vi "Helium Fridge Cool-Down - Copy.vi"() -> ()   [LabVIEW 2014]
uses:
  <vilib>/Analysis/8numeric.llb/1D Numeric Integration.vi
  <vilib>/express/express shared/transition.llb/Dynamic To Waveform Array.vi
  <vilib>/express/express signal manip/GetorSetDDTAttributes/Set DDT Attributes/SetT0.vi
  <vilib>/express/express shared/transition.llb/Waveform Array To Dynamic.vi
  <vilib>/express/express signal manip/GetorSetDDTAttributes/Set DDT Attributes/Set DDT Properties.xnode
  <vilib>/Analysis/NI_AALPro.lvlib
panel:
  out "Session Out 2":refnum<visa-resource-name>
  out "error out 2":errorcluster {"code" format="%.0x"}
  out "token":dbl
  in  "error in 2":errorcluster {"code" format="%.0x"}
  in  "Session In 2":refnum<visa-resource-name>="HPSIGGEN"
  in  "Depth/Div Submit":bool
  out "Depth/Div (kHz)":dbl
  in  "Cent. Frq. Submit":bool
  out "Session Out":refnum<visa-resource-name>
  out "error out":errorcluster {"code" format="%.0x"}
  out "Central Frequency":dbl
  in  "error in":errorcluster {"code" format="%.0x"}
  in  "Session In":refnum<visa-resource-name>="HPSIGGEN"
  out "Cent. Freq. (MHz)":dbl
  out "Temp 2":bool
  out "Temperature Strip Chart":dynamicdata(graph)
  in  "TC Points/Measurement":dbl=20.0
  out "NMR":bool
  out "NMR Temp Error":bool
  out "Q Meter Temp":dynamicdata(graph)
  out "Zeroed Array":dbl[](array[numeric])
  out "Fit X values":dbl[](array[numeric])
  in  "Left wing 2":dbl
  in  "Right wing 2":dbl
  in  "Right wing":dbl
  in  "Left wing":dbl
  out "Fit":dbl[](array[numeric])
  in  "Submit":bool
  out "Is Flashing":bool
  in  "Error Beat":bool
  in  "Clear":bool
  in  "Comment":string
  out "Heartbeat":bool
  out "Most Recent Error":string
  out "Baseline Subtracted Integral vs. Time":dbl(graph)
  out "Time of Last Baseline":string
  out "Baseline":dbl[](array[numeric])
  in  "Baseline Subtract":bool
  in  "Get Baseline":bool
  out "Recording":bool
  out "Time of Last Recording":string
  in  "Record \nNMR Sweeps":bool
  in  "Depth/Div\n(MHz)":dbl=10.0
  in  "Central Freq. \n(MHz)":dbl=13.0
  in  "stop (F)":bool caption="Triangle Wave"
  in  "Triangle Wave\nRate (Hz)":dbl=0.3
  out "Time Elapsed \nDuring Sweeps (s)":dbl
  out "Lab Time":string
  out "Most Recent Error (NMR)":string
  out "Last Sweep Start Time":string
  out "Most Recent Error (Temp)":string
  out "Last Measurement Taken":string
  out "VI Start Time":string
  in  "Time Between\nTemp Ponts (s)":dbl=30.0
  out "Temp":bool
  out "NMR":bool
  in  "stop":bool
  out "Input Triangle Wave":dynamicdata(graph)
  out "Modulator":dynamicdata(graph)
  out "NMR":cluster{"Y":dbl[], "Y":dbl[]}[](graph)
  in  "# of Sweeps":dbl=1.0
  out "Resistance Strip Chart":dynamicdata(graph)
  in  "Heartbeat":bool
  in  "Temp Strip Chart":bool
  out "Errors":bool
  in  "Silence Flashing":bool
  # "Initialization and Logic Controls -- DO NOT TOUCH!!"
  # "Caitlyn's Work"
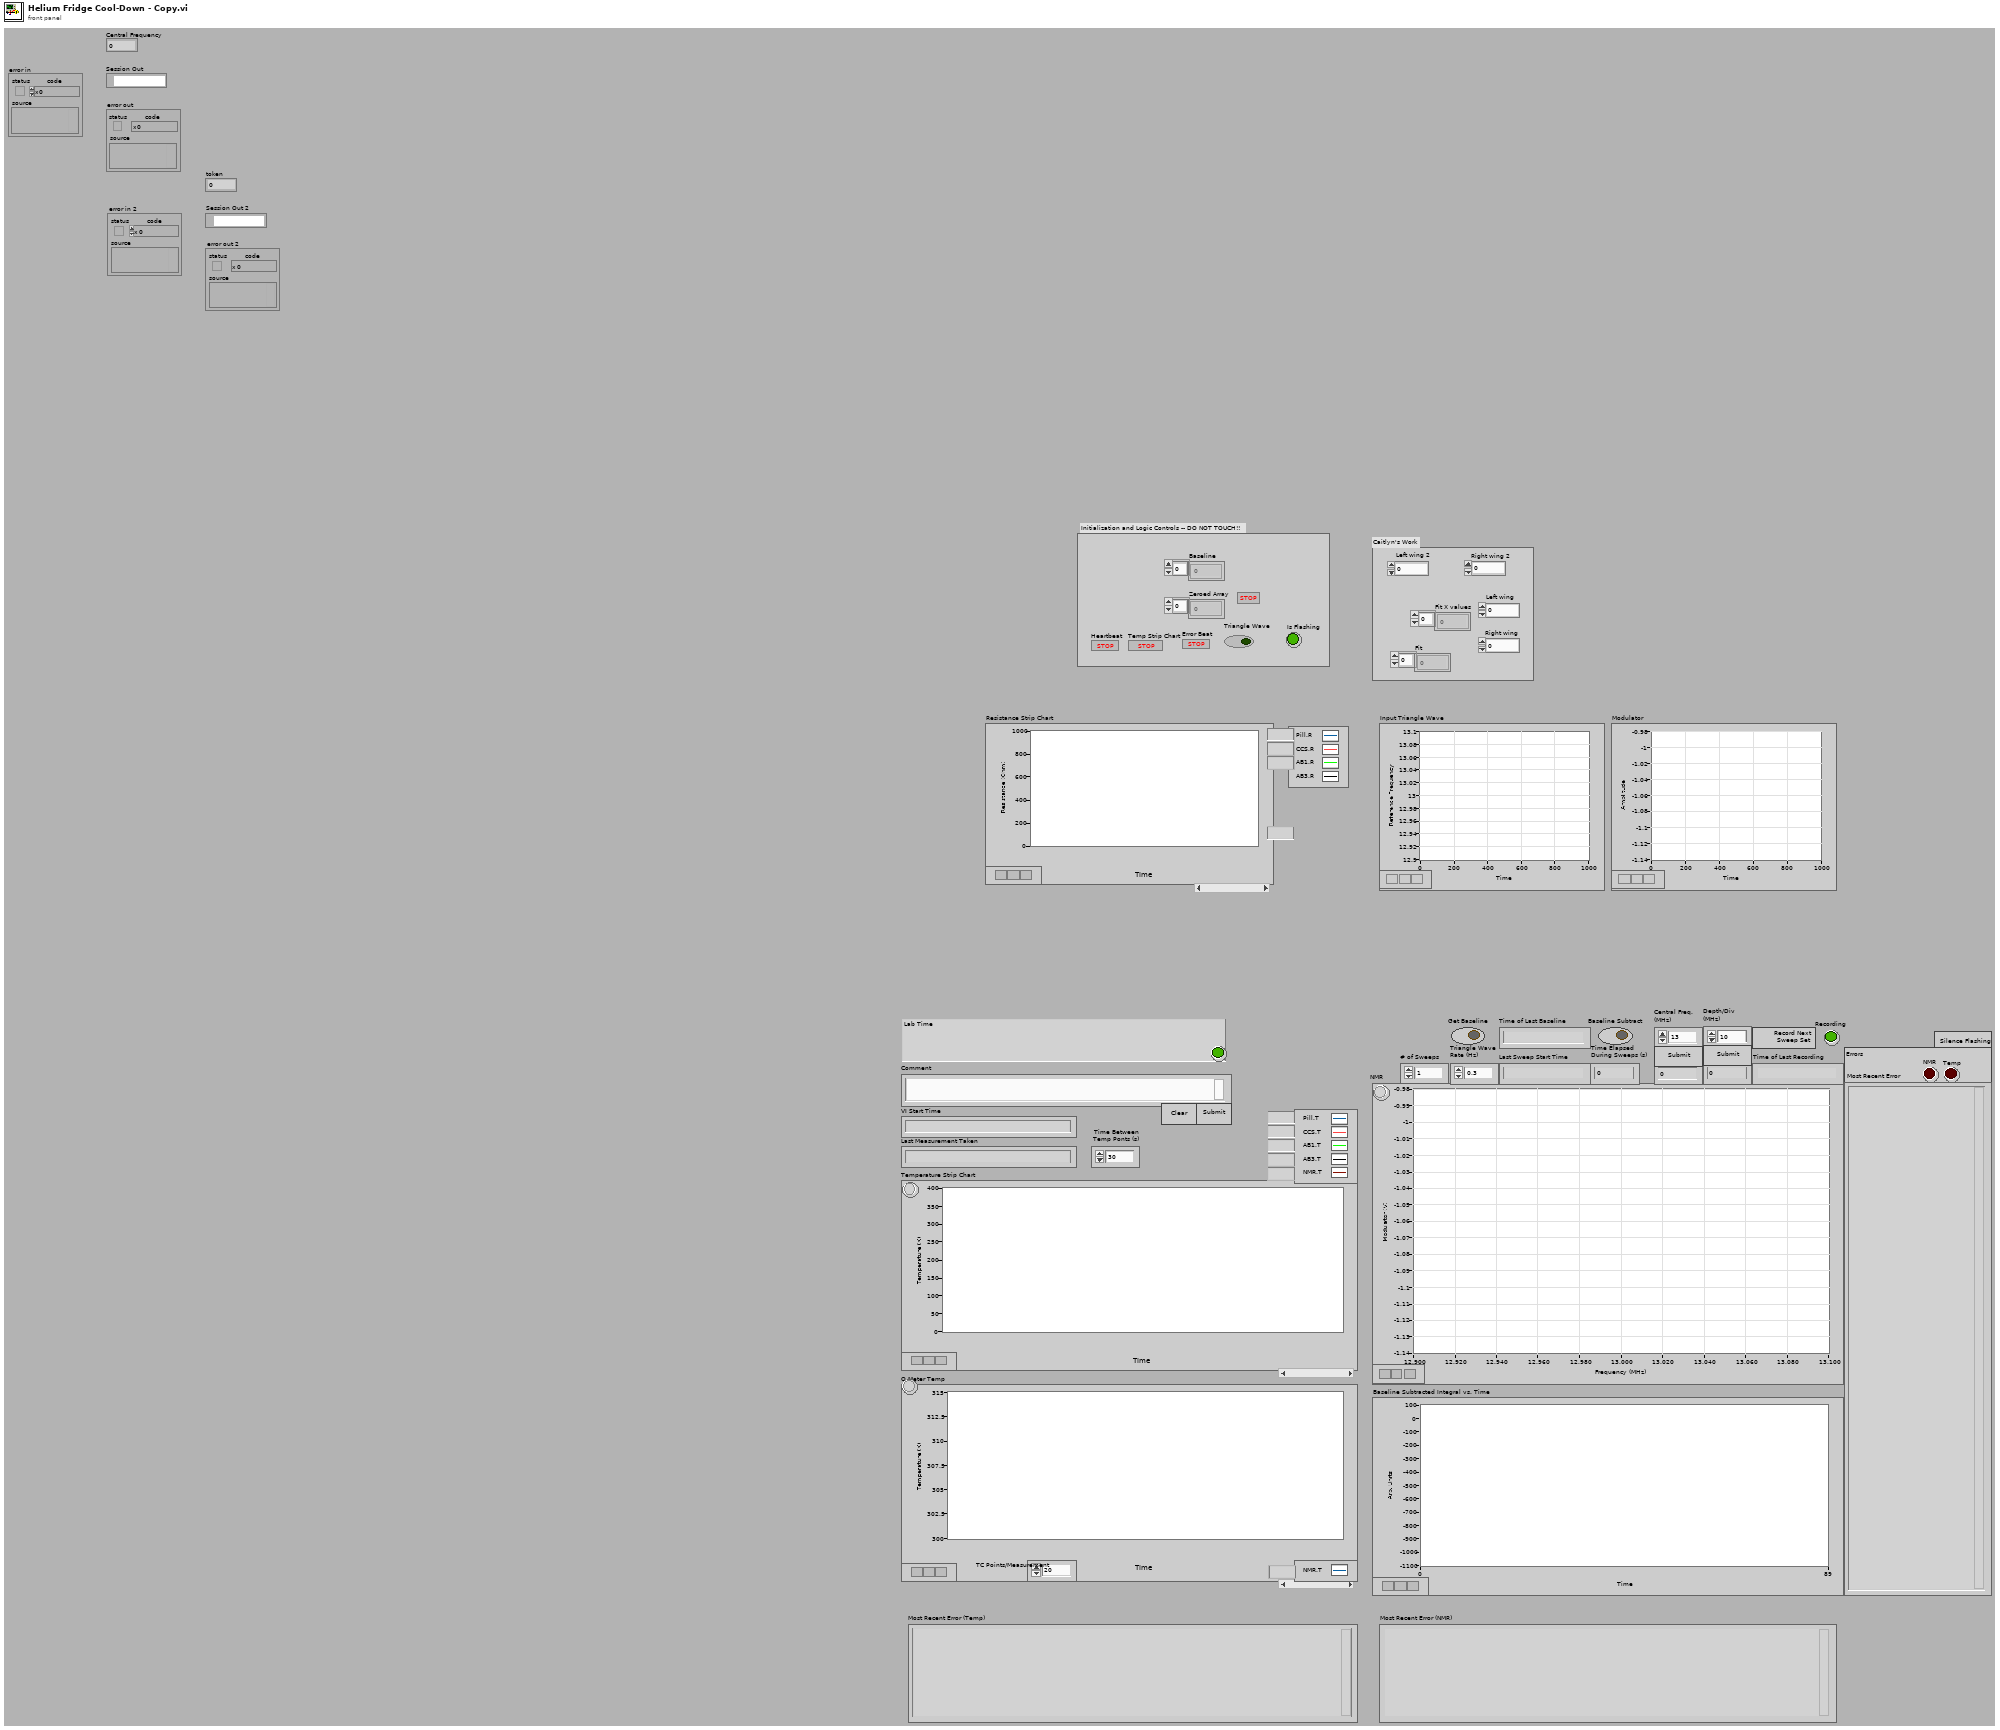
[diagram p1: front panel]
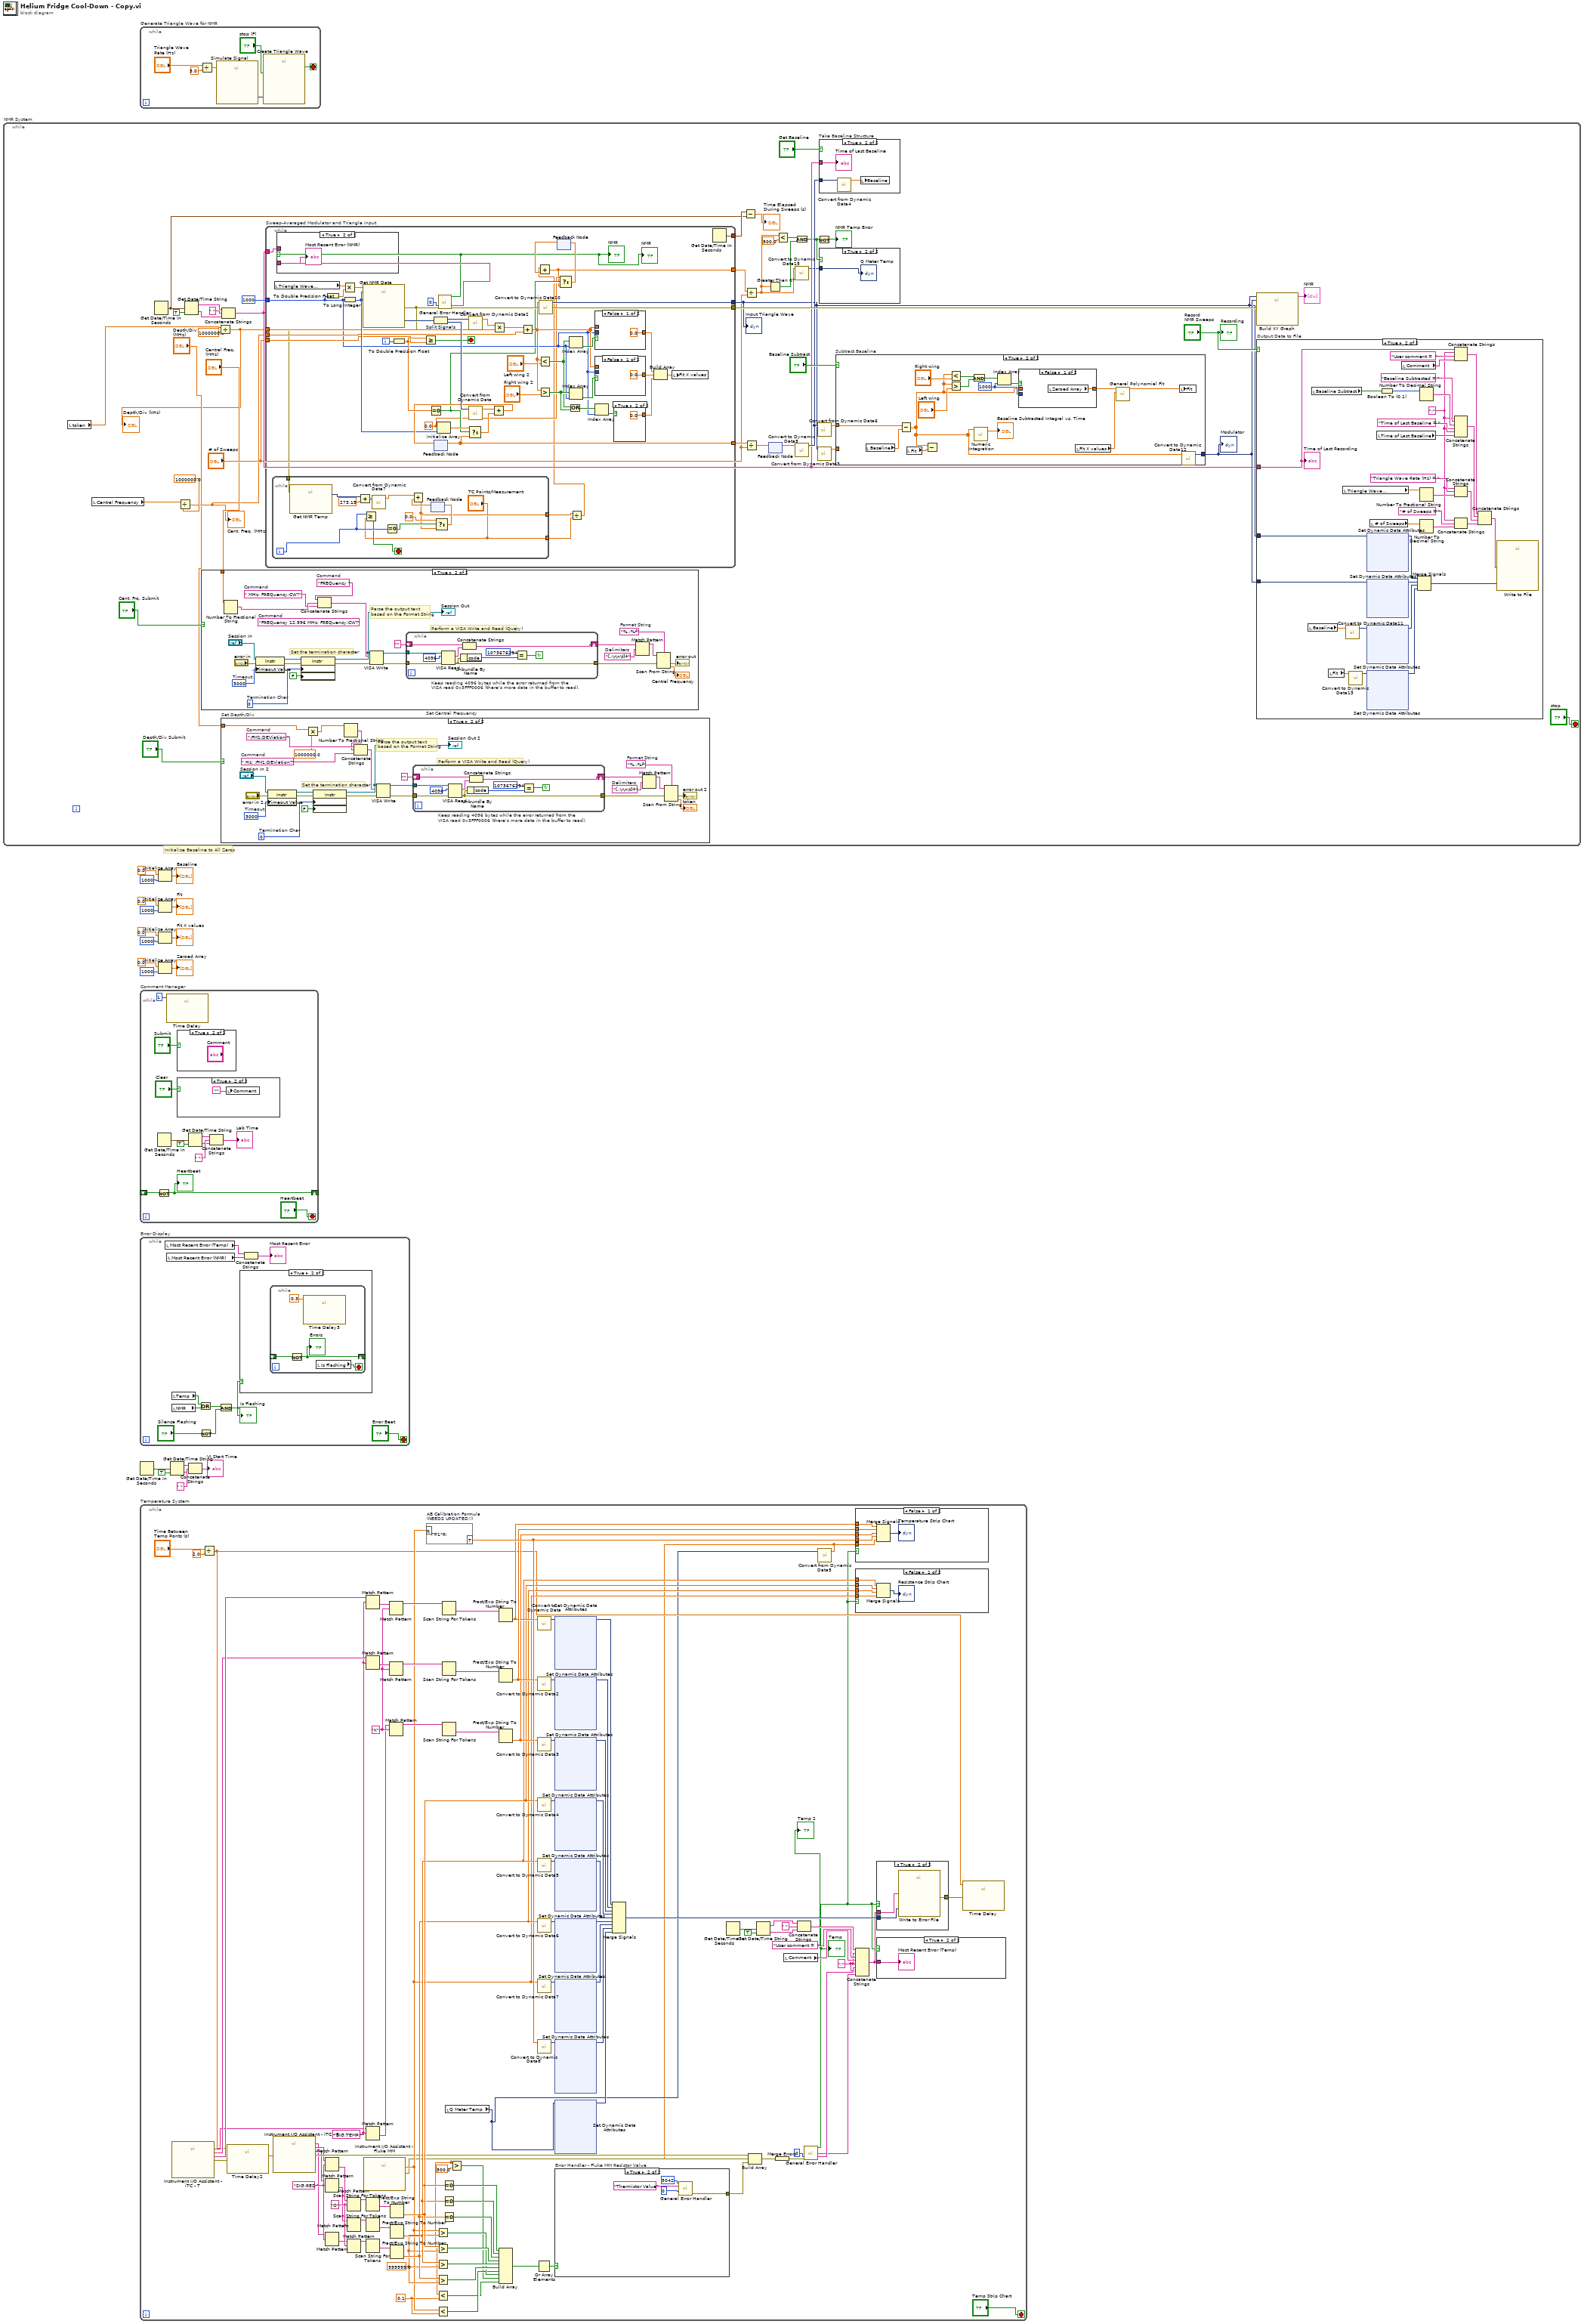
[diagram p0: block diagram]
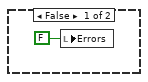
[diagram p2: hidden frame]
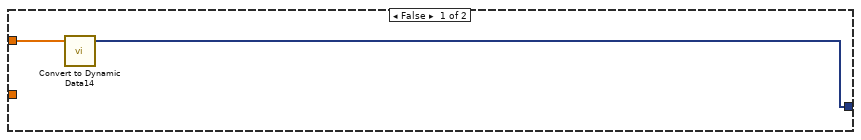
[diagram p6: hidden frame]
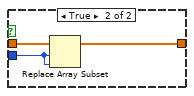
[diagram p7: hidden frame]
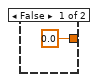
[diagram p10: hidden frame]
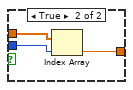
[diagram p11: hidden frame]
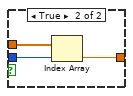
[diagram p12: hidden frame]
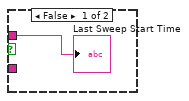
[diagram p13: hidden frame]
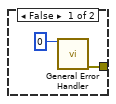
[diagram p16: hidden frame]
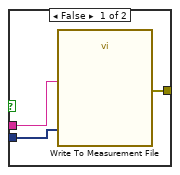
[diagram p19: hidden frame]
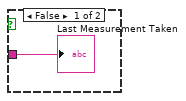
[diagram p20: hidden frame]
diagram:
  # "Initialize Baseline to All Zeros"
  n1 = while "NMR System" {
    stop <- "stop" stop-if-true
    n2 = local read "token"() -> (w20:dbl)
    n3 = local read "Central Frequency"() -> (w25:dbl)
    n4 = Get Date/Time In Seconds() -> (seconds since 1Jan1904=w49:timestamp)
    n5 = Divide(x=w25, y=1000000.0) -> (x/y=w23:dbl)
    "Cent. Freq. (MHz)" <- w23
    n6 = Get Date/Time String(seconds (now)=w49, want seconds? (F)=TRUE) -> (date string=w52:string, time string=w54:string)  [unwired: 1 in]
    n7 = case "Set Central Frequency" shown="True" "Cent. Frq. Submit" {
      tunnel: "Central Freq. \n(MHz)" -> [_ w100]
      frame False {
      }
      frame True {
        w98 = " MHz; FREQuency:CW?"  # Command
        w101 = "FREQuency "  # Command
        w119 = "[,;\r\n\t]+"  # Delimiters
        w116 = "%.;%f"  # Format String
        (unwired) "FREQuency 12.996 MHz; FREQuency:CW?"  # Command
        w107 = u8 0  # Termination Char
        w102 = u32 3000  # Timeout
        # "Parse the output text based on the Format String"
        # "Perform a VISA Write and Read (Query)"
        # "Keep reading 4096 bytes while the error returned from the\nVISA read 0x3FFF0006 (there's more data in the buffer to read)."
        # "Set the termination character"
        n8 = Number To Fractional String(number=w100) -> (F-format string=w99:string)  [unwired: 3 in]
        n9 = property class="Instr"(reference="Session In", error in="error in", "General Settings:Timeout Value"=w102) -> (reference out=w108:refnum<visa-resource-name>, error out=w105:errorcluster)
        n10 = property class="Instr"(reference=w108, error in=w105, "Message Based Settings:Termination Character"=w107, "Message Based Settings:Termination Character Enable"=FALSE ("enable")) -> (reference out=w120:refnum<visa-resource-name>, error out=w106:errorcluster)
        "Session Out" <- w120
        n11 = Concatenate Strings(w101, w99, w98) -> (w97:string)
        n12 = VISA Write(VISA resource name=w120, write buffer=w97, error in (no error)=w106) -> (VISA resource name out=w110:refnum<visa-resource-name>, error out=w111:errorcluster)  [unwired: 1 out]
        n13 = while {
          tunnel: w110 -> [w127]
          shift-right: [w121] -> w114
          shift-left: "" -> [w126]
          tunnel: w111 -> [w124]
          tunnel: [w123] -> w112
          stop <- w122 continue-if-true
          n14 = VISA Read(VISA resource name=w127, byte count=u32 4096 ("byte count (0)"), error in (no error)=w124) -> (read buffer=w125:string, error out=w123:errorcluster)  [unwired: 2 out]
          n15 = Unbundle By Name(w123) -> ("code"=w129:i32)
          n16 = Concatenate Strings(w126, w125) -> (w121:string)
          n17 = Equal?(x=1073676294, y=w129) -> (x = y?=w122:bool)
        }
        n18 = Match Pattern(string=w114, regular expression=w119) -> (before substring=w115:string)  [unwired: 1 in, 3 out]
        n19 = Scan From String(format string=w116, input string=w115, error in=w112) -> (error out=→"error out":errorcluster, output 1=→"Central Frequency":dbl)  [unwired: 2 in, 2 out]
      }
    }
    n20 = Divide(x=w20, y=1000000.0) -> (x/y=w19:dbl)
    "Depth/Div (kHz)" <- w19
    n21 = case "Set Depth/Div" shown="True" "Depth/Div Submit" {
      tunnel: "Depth/Div\n(MHz)" -> [_ w62]
      frame False {
      }
      frame True {
        w64 = " Hz; :FM1:DEViation?"  # Command
        w69 = "[,;\r\n\t]+"  # Delimiters
        w72 = "%.;%f"  # Format String
        w66 = ":FM1:DEViation "  # Command
        w81 = u8 0  # Termination Char
        w86 = u32 3000  # Timeout
        # "Parse the output text based on the Format String"
        # "Perform a VISA Write and Read (Query)"
        # "Keep reading 4096 bytes while the error returned from the\nVISA read 0x3FFF0006 (there's more data in the buffer to read)."
        # "Set the termination character"
        n22 = property class="Instr"(reference="Session In 2", error in="error in 2", "General Settings:Timeout Value"=w86) -> (reference out=w80:refnum<visa-resource-name>, error out=w83:errorcluster)
        n23 = Multiply(x=w62, y=1000000.0) -> (x*y=w61:dbl)
        n24 = property class="Instr"(reference=w80, error in=w83, "Message Based Settings:Termination Character"=w81, "Message Based Settings:Termination Character Enable"=FALSE ("enable")) -> (reference out=w68:refnum<visa-resource-name>, error out=w82:errorcluster)
        "Session Out 2" <- w68
        n25 = Number To Fractional String(number=w61) -> (F-format string=w65:string)  [unwired: 3 in]
        n26 = Concatenate Strings(w66, w65, w64) -> (w67:string)
        n27 = VISA Write(VISA resource name=w68, write buffer=w67, error in (no error)=w82) -> (VISA resource name out=w78:refnum<visa-resource-name>, error out=w77:errorcluster)  [unwired: 1 out]
        n28 = while {
          tunnel: w78 -> [w93]
          shift-right: [w87] -> w74
          shift-left: "" -> [w92]
          tunnel: w77 -> [w90]
          tunnel: [w89] -> w76
          stop <- w88 continue-if-true
          n29 = VISA Read(VISA resource name=w93, byte count=u32 4096 ("byte count (0)"), error in (no error)=w90) -> (read buffer=w91:string, error out=w89:errorcluster)  [unwired: 2 out]
          n30 = Unbundle By Name(w89) -> ("code"=w95:i32)
          n31 = Concatenate Strings(w92, w91) -> (w87:string)
          n32 = Equal?(x=1073676294, y=w95) -> (x = y?=w88:bool)
        }
        n33 = Match Pattern(string=w74, regular expression=w69) -> (before substring=w73:string)  [unwired: 1 in, 3 out]
        n34 = Scan From String(format string=w72, input string=w73, error in=w76) -> (error out=→"error out 2":errorcluster, output 1=→"token":dbl)  [unwired: 2 in, 2 out]
      }
    }
    n35 = Concatenate Strings(w52, " ", w54) -> (w40:string)
    n36 = while "Sweep-Averaged Modulator and Triangle Input" {
      tunnel: "# of Sweeps" -> [w285]
      tunnel: 1000 -> [w276]
      tunnel: [w302] -> w57
      tunnel: w40 -> [w298]
      tunnel: [w297] -> w50
      tunnel: [w295] -> w47
      tunnel: w19 -> [w289]
      tunnel: w23 -> [w287]
      tunnel: [w286] -> w39
      tunnel: [w266] -> w28
      i -> [w308]
      stop <- w301 stop-if-true
      w269 = 0.0
      n37 = local read "Triangle Wave\nRate (Hz)"() -> (w294:dbl)
      n38 = To Double Precision Float(number=w276) -> (double precision float=w292:dbl)
      n39 = Multiply(x=w294, y=w292) -> (x*y=w296:dbl)
      n40 = To Long Integer(number=w276) -> (32bit integer=w293:i32)
      n41 = call "Get NMR Data"("rate"=w296, "number of samples"=w293) -> ("data"=w310:dynamicdata, "error out"=w261:errorcluster)  [unwired: 15 in, 1 out]
      n42 = while {
        tunnel: ["TC Points/Measurement"] -> w264
        tunnel: [w315] -> w263
        tunnel: w261 -> [w314]
        i -> [w313]
        stop <- w312 stop-if-true
        n43 = call "Get NMR Temp"("error in"=w314) -> ("data"=w317:dynamicdata)  [unwired: 16 in, 2 out]
        n44 = Add(x=w317, y=273.15) -> (x+y=w316:dynamicdata)
        n45 = Greater Or Equal?(x=w313, y="TC Points/Measurement") -> (x >= y?=w312:bool)
        n46 = call "Convert from Dynamic Data7"("Dynamic Data Type"=w316) -> ("Scalar"=w319:dbl)  [unwired: 3 in]
        n47 = Equal To 0?(x=w313) -> (x = 0?=w320:bool)
        n48 = feedback #1() -> (w322:dbl)  [unwired: 1 in]
        n49 = Add(x=w319, y=w322) -> (x+y=w315:dbl)
        n50 = Select(t=0.0, s=w320, f=w315) -> (s? t:f=w321:dbl)
        n51 = feedback-in #1(w321) -> ()
      }
      n52 = To Double Precision Float(number=w308) -> (double precision float=w307:dbl)
      n53 = Greater Or Equal?(x=w307, y=w285) -> (x >= y?=w301:bool)
      n54 = Equal To 0?(x=w307) -> (x = 0?=w270:bool)
      n55 = Split Signals(w310) -> (w291:dynamicdata, w309:dynamicdata)  [unwired: 2 in]
      n56 = feedback #2() -> (w302:dbl[])  [unwired: 1 in]
      n57 = Initialize Array(w269, w293) -> (w305:dbl[])
      n58 = call <vilib>:"General Error Handler.vi"("type of dialog (OK msg:1)"=0, "error in (no error)"=w261) -> ("error?"=w265:bool, "message"=w300:string, "error out"=w295:errorcluster)  [unwired: 9 in, 2 out]
      "NMR" <- w265
      "NMR" <- w265
      n59 = case shown="True" w265 {
        tunnel: w300 -> [_ w335]
        tunnel: w298 -> [w334 _]
        frame False {
          "Last Sweep Start Time" <- w334
        }
        frame True {
          "Most Recent Error (NMR)" <- w335
        }
      }
      n60 = call "Convert from Dynamic Data2"("Dynamic Data Type"=w291) -> ("Array"=w290:dbl[])  [unwired: 3 in]
      n61 = call "Convert from Dynamic Data"("Dynamic Data Type"=w309) -> ("Array"=w304:dbl[])  [unwired: 3 in]
      n62 = Select(t=w305, s=w270, f=w302) -> (s? t:f=w306:dbl[])
      n63 = Add(x=w304, y=w306) -> (x+y=w303:dbl[])
      n64 = feedback-in #2(w303) -> ()
      n65 = Multiply(x=w290, y=w289) -> (x*y=w288:dbl[])
      n66 = Add(x=w288, y=w287) -> (x+y=w282:dbl[])
      n67 = Less?(x=w282, y="Left wing 2") -> (x < y?=w278:bool[])
      n68 = Greater?(x=w282, y="Right wing 2") -> (0:w279:bool[])
      n69 = call "Convert to Dynamic Data10"("Array"=w282) -> ("Dynamic Data Type"=w286:dynamicdata)  [unwired: 3 in]
      n70 = feedback #3() -> (w267:dbl)  [unwired: 1 in]
      n71 = Or(x=w278, y=w279) -> (x .or. y?=w277:bool[])
      n72 = Index Array(array=w278, index=w276) -> (element=w284:bool)
      n73 = Index Array(array=w279, index=w276) -> (element=w283:bool)
      n74 = Divide(x=w263, y=w264) -> (x/y=w262:dbl)
      n75 = Add(x=w262, y=w267) -> (x+y=w266:dbl)
      n76 = Select(t=w269, s=w270, f=w266) -> (s? t:f=w268:dbl)
      n77 = feedback-in #3(w268) -> ()
      n78 = case shown="False" w284 {
        tunnel: w282 -> [_ w333]
        tunnel: w276 -> [_ w332]
        tunnel: [0.0 w331] -> w280
        frame False {
        }
        frame True {
          n79 = Index Array(array=w333, index=w332) -> (element=w331:dbl)
        }
      }
      n80 = case shown="False" w283 {
        tunnel: w282 -> [_ w329]
        tunnel: w276 -> [_ w328]
        tunnel: [0.0 w327] -> w281
        frame False {
        }
        frame True {
          n81 = Index Array(array=w329, index=w328) -> (element=w327:dbl)
        }
      }
      n82 = Index Array(array=w277, index=w276) -> (element=w275:bool)
      n83 = case shown="True" w275 {
        tunnel: [0.0 0.0] -> w274
        frame False {
        }
        frame True {
        }
      }
      n84 = Build Array(w280, w281, w274) -> (w271:dbl[])
      n85 = local write "Fit X values"(w271) -> ()
      n86 = Get Date/Time In Seconds() -> (seconds since 1Jan1904=w297:timestamp)
    }
    "Input Triangle Wave" <- w39
    n87 = Subtract(x=w50, y=w49) -> (x-y=→"Time Elapsed \nDuring Sweeps (s)":dbl)
    n88 = Divide(x=w28, y="# of Sweeps") -> (x/y=w29:dbl)
    n89 = Divide(x=w57, y="# of Sweeps") -> (x/y=w56:dbl[])
    n90 = Greater Than 0?(x=w29) -> (x > 0?=w36:bool)
    n91 = feedback-in #4(w56) -> ()
    n92 = feedback #4() -> (w55:dbl[])  [unwired: 1 in]
    n93 = Less?(x=w29, y=500.0) -> (x < y?=w33:bool)
    n94 = And(x=w33, y=w36) -> (x .and. y?=w35:bool)
    n95 = call "Convert to Dynamic Data15"("Double"=w29) -> ("Dynamic Data Type"=w31:dynamicdata)  [unwired: 3 in]
    n96 = call "Convert to Dynamic Data9"("Array"=w55) -> ("Dynamic Data Type"=w42:dynamicdata)  [unwired: 3 in]
    n97 = Not(x=w35) -> (.not. x?=→"NMR Temp Error":bool)
    n98 = call "Convert from Dynamic Data6"("Dynamic Data Type"=w42) -> ("Array"=w37:dbl[])  [unwired: 3 in]
    n99 = call "Convert from Dynamic Data3"("Dynamic Data Type"=w39) -> ("Array"=w38:dbl[])  [unwired: 3 in]
    n100 = case "Take Baseline Structure" shown="True" "Get Baseline" {
      tunnel: w42 -> [_ w156]
      tunnel: w40 -> [_ w154]
      frame False {
      }
      frame True {
        n101 = call "Convert from Dynamic Data4"("Dynamic Data Type"=w156) -> ("Array"=w155:dbl[])  [unwired: 3 in]
        n102 = local write "Baseline"(w155) -> ()
        "Time of Last Baseline" <- w154
      }
    }
    n103 = case shown="True" w35 {
      tunnel: w31 -> [_ w131]
      frame False {
      }
      frame True {
        "Q Meter Temp" <- w131
      }
    }
    n104 = case "Subtract Baseline" shown="True" "Baseline Subtract" {
      tunnel: w37 -> [w133 w149]
      tunnel: [w132 w148] -> w41
      tunnel: w38 -> [_ _]
      frame False {
        n105 = call "Convert to Dynamic Data14"("Array"=w133) -> ("Dynamic Data Type"=w132:dynamicdata)  [unwired: 3 in]
      }
      frame True {
        w138 = 1000
        n106 = local read "Baseline"() -> (w146:dbl[])
        n107 = Subtract(x=w149, y=w146) -> (x-y=w134:dbl[])
        n108 = local read "Fit"() -> (w145:dbl[])
        n109 = Subtract(x=w134, y=w145) -> ()  [unwired: 1 out]
        n110 = Less?(x=w134, y="Right wing") -> (x < y?=w142:bool[])
        n111 = Greater?(x=w134, y="Left wing") -> (0:w141:bool[])
        n112 = And(x=w142, y=w141) -> (x .and. y?=w140:bool[])
        n113 = call-poly <vilib>:"Numeric Integration.vi"("Input Array"=w134) -> ("result"=→"Baseline Subtracted Integral vs. Time":dbl)  [unwired: 2 in, 1 out]
        n114 = Index Array(array=w140, index=w138) -> (element=w139:bool)
        n115 = case shown="False" w139 {
          tunnel: w134 -> [_ w153]
          tunnel: w138 -> [_ w151]
          tunnel: [w150 w152] -> w137
          frame False {
            n116 = local read "Zeroed Array"() -> (w150:dbl[])
          }
          frame True {
            n117 = Replace Array Subset(array=w153, new element=w151, index=w151) -> (w152:dbl[])
          }
        }
        n118 = local read "Fit X values"() -> (w135:dbl[])
        n119 = call <vilib>:"General Polynomial Fit.vi"("Y"=w137, "X"=w135) -> ("Best Polynomial Fit"=w136:dbl[])  [unwired: 10 in, 3 out]
        n120 = local write "Fit"(w136) -> ()
        n121 = call "Convert to Dynamic Data12"("Array"=w134) -> ("Dynamic Data Type"=w148:dynamicdata)  [unwired: 3 in]
      }
    }
    "Modulator" <- w41
    n122 = call "Build XY Graph"("error in (no error)"=w47, "Y Input"=w41, "X Input"=w39) -> ("XY Graph"=→"NMR":cluster{"Y":dbl[], "Y":dbl[]}[])  [unwired: 7 in, 1 out]
    n123 = case "Output Data to File" shown="True" "Record \nNMR Sweeps" {
      tunnel: w40 -> [_ w177]
      tunnel: w41 -> [_ w184]
      tunnel: w39 -> [_ w183]
      frame False {
      }
      frame True {
        w161 = ";"
        n124 = local read "Baseline"() -> (w182:dbl[])
        n125 = local read "Baseline Subtract"() -> (w179:bool)
        n126 = local read "Fit"() -> (w160:dbl[])
        n127 = local read "Triangle Wave\nRate (Hz)"() -> (w180:dbl)
        n128 = call "Convert to Dynamic Data11"("Array"=w182) -> ("Dynamic Data Type"=w181:dynamicdata)  [unwired: 3 in]
        n129 = call "Convert to Dynamic Data13"("Array"=w160) -> ("Dynamic Data Type"=w159:dynamicdata)  [unwired: 3 in]
        n130 = xnode "Set Dynamic Data Attributes"("Signals In"=w183) -> ("Signals Out"=w188:dynamicdata)  [unwired: 4 in, 1 out]
        n131 = xnode "Set Dynamic Data Attributes"("Signals In"=w184) -> ("Signals Out"=w186:dynamicdata)  [unwired: 4 in, 1 out]
        n132 = xnode "Set Dynamic Data Attributes"("Signals In"=w181) -> ("Signals Out"=w158:dynamicdata)  [unwired: 4 in, 1 out]
        n133 = xnode "Set Dynamic Data Attributes"("Signals In"=w159) -> ("Signals Out"=w157:dynamicdata)  [unwired: 4 in, 1 out]
        n134 = local read "# of Sweeps"() -> (w185:dbl)
        n135 = local read "Time of Last Baseline"() -> (w166:string)
        n136 = Boolean To (0,1)(Boolean=w179) -> (0, 1=w178:i16)
        n137 = local read "Comment"() -> (w175:string)
        n138 = Merge Signals(w188, w186, w158, w157) -> (w187:dynamicdata)
        n139 = Number To Decimal String(number=w178) -> (decimal integer string=w171:string)  [unwired: 1 in]
        n140 = Number To Fractional String(number=w180) -> (F-format string=w169:string)  [unwired: 3 in]
        n141 = Number To Decimal String(number=w185) -> (decimal integer string=w173:string)  [unwired: 1 in]
        n142 = Concatenate Strings(w177, w161, "User comment =  ", w175) -> (w168:string)
        n143 = Concatenate Strings(w161, "Baseline Subtracted = ", w171, w161, "Time of Last Baseline = ", w166) -> (w165:string)
        n144 = Concatenate Strings(w161, "Triangle Wave Rate (Hz) = ", w169) -> (w164:string)
        n145 = Concatenate Strings(w161, "# of Sweeps = ", w173) -> (w163:string)
        n146 = Concatenate Strings(w168, w165, w164, w163) -> (w162:string)
        n147 = call "Write to File"("Signals"=w187, "Comment"=w162) -> ()  [unwired: 15 in, 3 out]
        "Time of Last Recording" <- w177
      }
    }
    "Recording" <- "Record \nNMR Sweeps"
  }
  n148 = while "Generate Triangle Wave for NMR" {
    stop <- w340 stop-if-true
    n149 = Divide(x="Triangle Wave\nRate (Hz)", y=5.0) -> (x/y=w336:dbl)
    n150 = call "Simulate Signal"("Frequency"=w336) -> ("Triangle"=w339:dynamicdata)  [unwired: 13 in, 1 out]
    n151 = call "Create Triangle Wave"("data"=w339, "stop (F)"="stop (F)") -> ("stopped"=w340:bool)  [unwired: 15 in, 2 out]
  }
  n152 = while "Comment Manager" {
    shift-right: [w350] -> _
    shift-left: _ -> [w353]
    stop <- "Heartbeat" stop-if-true
    n153 = Not(x=w353) -> (.not. x?=w350:bool)
    "Heartbeat" <- w350
    n154 = Get Date/Time In Seconds() -> (seconds since 1Jan1904=w348:timestamp)
    n155 = call "Time Delay"("Delay Time (s)"=1) -> ()  [unwired: 10 in, 1 out]
    n156 = case shown="True" "Submit" {
      frame False {
      }
      frame True {
      }
    }
    n157 = case shown="True" "Clear" {
      frame False {
      }
      frame True {
        n158 = local write "Comment"("") -> ()
      }
    }
    n159 = Get Date/Time String(seconds (now)=w348, want seconds? (F)=TRUE) -> (date string=w347:string, time string=w345:string)  [unwired: 1 in]
    n160 = Concatenate Strings(w347, " ", w345) -> (→"Lab Time":string)
  }
  n161 = while "Error Display" {
    stop <- "Error Beat" stop-if-true
    n162 = local read "Most Recent Error (Temp)"() -> (w355:string)
    n163 = local read "Most Recent Error (NMR)"() -> (w356:string)
    n164 = local read "Temp"() -> (w364:bool)
    n165 = local read "NMR"() -> (w363:bool)
    n166 = Or(x=w364, y=w363) -> (x .or. y?=w361:bool)
    n167 = Not(x="Silence Flashing") -> (.not. x?=w359:bool)
    n168 = And(x=w361, y=w359) -> (x .and. y?=w358:bool)
    "Is Flashing" <- w358
    n169 = case shown="True" w358 {
      frame False {
        n170 = local write "Errors"(FALSE) -> ()
      }
      frame True {
        n171 = while {
          shift-right: [w367] -> _
          shift-left: _ -> [w369]
          stop <- w366 stop-if-true
          n172 = Not(x=w369) -> (.not. x?=w367:bool)
          "Errors" <- w367
          n173 = call "Time Delay3"("Delay Time (s)"=0.3) -> ()  [unwired: 10 in, 1 out]
          n174 = local read "Is Flashing"() -> (w366:bool)
        }
      }
    }
    n175 = Concatenate Strings(w355, w356) -> (→"Most Recent Error":string)
  }
  n176 = Get Date/Time In Seconds() -> (seconds since 1Jan1904=w17:timestamp)
  n177 = while "Temperature System" {
    stop <- "Temp Strip Chart" stop-if-true
    w378 = ";"
    w374 = 0.1
    w400 = 999999.0
    w436 = "O"
    w437 = "SIG:RES:"
    w443 = "SIG:TEMP:"
    w442 = "K"
    n178 = call "Instrument I/O Assistant - iTC - T"() -> ("AB1.T"=w441:string, "CCS.T"=w446:string, "Pill.T"=w449:string, "error out"=w391:errorcluster)  [unwired: 23 in, 1 out]
    n179 = Divide(x="Time Between\nTemp Ponts (s)", y=2.0) -> (x/y=w386:dbl)
    n180 = call "Time Delay2"("error in (no error)"=w391, "Delay Time (s)"=w386) -> ("error out"=w392:errorcluster)  [unwired: 9 in]
    n181 = call "Instrument I/O Assistant - iTC - R"("error in"=w392) -> ("AB1.R"=w388:string, "CCS.R"=w389:string, "Pill.R"=w390:string, "error out"=w393:errorcluster)  [unwired: 22 in, 1 out]
    n182 = Match Pattern(string=w389, regular expression=w437) -> (after substring=w435:string)  [unwired: 1 in, 3 out]
    n183 = Match Pattern(string=w390, regular expression=w437) -> (after substring=w434:string)  [unwired: 1 in, 3 out]
    n184 = Match Pattern(string=w388, regular expression=w437) -> (after substring=w433:string)  [unwired: 1 in, 3 out]
    n185 = Match Pattern(string=w435, regular expression=w436) -> (before substring=w432:string)  [unwired: 1 in, 3 out]
    n186 = Match Pattern(string=w434, regular expression=w436) -> (before substring=w431:string)  [unwired: 1 in, 3 out]
    n187 = Match Pattern(string=w433, regular expression=w436) -> (before substring=w430:string)  [unwired: 1 in, 3 out]
    n188 = call "Instrument I/O Assistant - Fluke MM"() -> ("AB3.R"=w398:dbl, "error out"=w396:errorcluster)  [unwired: 25 in, 1 out]
    n189 = Match Pattern(string=w449, regular expression=w443) -> (after substring=w448:string)  [unwired: 1 in, 3 out]
    n190 = Match Pattern(string=w446, regular expression=w443) -> (after substring=w445:string)  [unwired: 1 in, 3 out]
    n191 = Match Pattern(string=w441, regular expression=w443) -> (after substring=w440:string)  [unwired: 1 in, 3 out]
    n192 = Scan String For Tokens(9:w432) -> (1:w429:string)  [unwired: 5 in, 3 out]
    n193 = Scan String For Tokens(9:w431) -> (1:w428:string)  [unwired: 5 in, 3 out]
    n194 = Scan String For Tokens(9:w430) -> (1:w427:string)  [unwired: 5 in, 3 out]
    n195 = Match Pattern(string=w448, regular expression=w442) -> (before substring=w447:string)  [unwired: 1 in, 3 out]
    n196 = Match Pattern(string=w445, regular expression=w442) -> (before substring=w444:string)  [unwired: 1 in, 3 out]
    n197 = Match Pattern(string=w440, regular expression=w442) -> (before substring=w439:string)  [unwired: 1 in, 3 out]
    n198 = Fract/Exp String To Number(string=w429) -> (number=w406:dbl)  [unwired: 3 in, 1 out]
    n199 = Fract/Exp String To Number(string=w428) -> (number=w405:dbl)  [unwired: 3 in, 1 out]
    n200 = Fract/Exp String To Number(string=w427) -> (number=w404:dbl)  [unwired: 3 in, 1 out]
    n201 = formula code="T=1*R;" "AB Calibration Formula\n(NEEDS UPDATED!!)"("R"=w398) -> ("T"=w417:dbl)
    n202 = Greater?(x=w398, y=w400) -> (0:w399:bool)
    n203 = Greater?(x=w406, y=w400) -> (0:w403:bool)
    n204 = Greater?(x=w405, y=w400) -> (0:w402:bool)
    n205 = Greater?(x=w404, y=w400) -> (0:w401:bool)
    n206 = Less?(x=w398, y=w374) -> (x < y?=w397:bool)
    n207 = Scan String For Tokens(9:w447) -> (1:w466:string)  [unwired: 5 in, 3 out]
    n208 = Scan String For Tokens(9:w444) -> (1:w464:string)  [unwired: 5 in, 3 out]
    n209 = Scan String For Tokens(9:w439) -> (1:w463:string)  [unwired: 5 in, 3 out]
    n210 = Equal To 0?(x=w406) -> (x = 0?=w414:bool)
    n211 = Equal To 0?(x=w405) -> (x = 0?=w413:bool)
    n212 = Equal To 0?(x=w404) -> (x = 0?=w412:bool)
    n213 = local read "Q Meter Temp"() -> (w371:dynamicdata)
    n214 = Fract/Exp String To Number(string=w466) -> (number=w408:dbl)  [unwired: 3 in, 1 out]
    n215 = Fract/Exp String To Number(string=w464) -> (number=w409:dbl)  [unwired: 3 in, 1 out]
    n216 = Fract/Exp String To Number(string=w463) -> (number=w407:dbl)  [unwired: 3 in, 1 out]
    n217 = call "Convert to Dynamic Data"("Double"=w408) -> ("Dynamic Data Type"=w457:dynamicdata)  [unwired: 3 in]
    n218 = call "Convert to Dynamic Data2"("Double"=w409) -> ("Dynamic Data Type"=w455:dynamicdata)  [unwired: 3 in]
    n219 = call "Convert to Dynamic Data3"("Double"=w407) -> ("Dynamic Data Type"=w454:dynamicdata)  [unwired: 3 in]
    n220 = call "Convert to Dynamic Data4"("Double"=w406) -> ("Dynamic Data Type"=w426:dynamicdata)  [unwired: 3 in]
    n221 = call "Convert to Dynamic Data5"("Double"=w405) -> ("Dynamic Data Type"=w425:dynamicdata)  [unwired: 3 in]
    n222 = call "Convert to Dynamic Data6"("Double"=w404) -> ("Dynamic Data Type"=w424:dynamicdata)  [unwired: 3 in]
    n223 = call "Convert to Dynamic Data7"("Double"=w398) -> ("Dynamic Data Type"=w420:dynamicdata)  [unwired: 3 in]
    n224 = call "Convert to Dynamic Data8"("Double"=w417) -> ("Dynamic Data Type"=w416:dynamicdata)  [unwired: 3 in]
    n225 = xnode "Set Dynamic Data Attributes"("Signals In"=w457) -> ("Signals Out"=w456:dynamicdata)  [unwired: 4 in, 1 out]
    n226 = xnode "Set Dynamic Data Attributes"("Signals In"=w455) -> ("Signals Out"=w453:dynamicdata)  [unwired: 4 in, 1 out]
    n227 = xnode "Set Dynamic Data Attributes"("Signals In"=w454) -> ("Signals Out"=w452:dynamicdata)  [unwired: 4 in, 1 out]
    n228 = xnode "Set Dynamic Data Attributes"("Signals In"=w426) -> ("Signals Out"=w423:dynamicdata)  [unwired: 4 in, 1 out]
    n229 = xnode "Set Dynamic Data Attributes"("Signals In"=w425) -> ("Signals Out"=w422:dynamicdata)  [unwired: 4 in, 1 out]
    n230 = xnode "Set Dynamic Data Attributes"("Signals In"=w424) -> ("Signals Out"=w421:dynamicdata)  [unwired: 4 in, 1 out]
    n231 = xnode "Set Dynamic Data Attributes"("Signals In"=w420) -> ("Signals Out"=w419:dynamicdata)  [unwired: 4 in, 1 out]
    n232 = xnode "Set Dynamic Data Attributes"("Signals In"=w416) -> ("Signals Out"=w415:dynamicdata)  [unwired: 4 in, 1 out]
    n233 = xnode "Set Dynamic Data Attributes"("Signals In"=w371) -> ("Signals Out"=w377:dynamicdata)  [unwired: 4 in, 1 out]
    n234 = Merge Signals(w456, w453, w452, w423, w422, w421, w419, w415, w377) -> (w451:dynamicdata)
    n235 = Get Date/Time In Seconds() -> (seconds since 1Jan1904=w462:timestamp)
    n236 = Get Date/Time String(seconds (now)=w462, want seconds? (F)=TRUE) -> (date string=w460:string, time string=w458:string)  [unwired: 1 in]
    n237 = local read "Comment"() -> (w383:string)
    n238 = Concatenate Strings(w460, " ", w458) -> (w379:string)
    n239 = call "Convert from Dynamic Data5"("Dynamic Data Type"=w371) -> ("Scalar"=w370:dbl)  [unwired: 3 in]
    n240 = Less?(x=w370, y=w374) -> (x < y?=w373:bool)
    n241 = Greater?(x=w370, y=500.0) -> (0:w375:bool)
    n242 = Build Array(w414, w413, w412, w403, w402, w401, w397, w399, w375, w373) -> (w411:bool[])
    n243 = Or Array Elements(Boolean array=w411) -> (logical OR=w410:bool)
    n244 = case "Error Handler - Fluke MM Resistor Value" shown="True" w410 {
      tunnel: [w485 w490] -> w395
      frame False {
        n245 = call <vilib>:"General Error Handler.vi"("[error code] (0)"=0) -> ("error out"=w485:errorcluster)  [unwired: 10 in, 4 out]
      }
      frame True {
        n246 = call <vilib>:"General Error Handler.vi"("[error code] (0)"=5042, "[error source] (\" \")"="Thermistor Value", "type of dialog (OK msg:1)"=0) -> ("error out"=w490:errorcluster)  [unwired: 8 in, 4 out]
      }
    }
    n247 = Build Array(w393, w396, w395) -> (w394:errorcluster[])
    n248 = Merge Errors(w394) -> (w418:errorcluster)
    n249 = call <vilib>:"General Error Handler.vi"("type of dialog (OK msg:1)"=0, "error in (no error)"=w418) -> ("error?"=w372:bool, "source out"=w380:string, "message"=w382:string)  [unwired: 9 in, 2 out]
    "Temp" <- w372
    "Temp 2" <- w372
    n250 = case shown="False" w372 {
      tunnel: w408 -> [w591 _]
      tunnel: w409 -> [w590 _]
      tunnel: w407 -> [w589 _]
      tunnel: w417 -> [w588 _]
      tunnel: w370 -> [w586 _]
      frame False {
        n251 = Merge Signals(w591, w590, w589, w588, w586) -> (→"Temperature Strip Chart":dynamicdata)
      }
      frame True {
      }
    }
    n252 = case shown="False" w372 {
      tunnel: w405 -> [w585 _]
      tunnel: w406 -> [w584 _]
      tunnel: w404 -> [w583 _]
      tunnel: w398 -> [w582 _]
      frame False {
        n253 = Merge Signals(w585, w584, w583, w582) -> (→"Resistance Strip Chart":dynamicdata)
      }
      frame True {
      }
    }
    n254 = Concatenate Strings(w379, w378, "User comment =  ", w383, w378, w382, w378, w380) -> (w381:string)
    n255 = case shown="True" w372 {
      tunnel: w451 -> [w594 w597]
      tunnel: w381 -> [w593 w596]
      tunnel: [w592 w595] -> w438
      frame False {
        n256 = call "Write To Measurement File"("Signals"=w594, "Comment"=w593) -> ("error out"=w592:errorcluster)  [unwired: 15 in, 2 out]
      }
      frame True {
        n257 = call "Write to Error File"("Signals"=w597, "Comment"=w596) -> ("error out"=w595:errorcluster)  [unwired: 15 in, 2 out]
      }
    }
    n258 = case shown="True" w372 {
      tunnel: w381 -> [w652 w653]
      frame False {
        "Last Measurement Taken" <- w652
      }
      frame True {
        "Most Recent Error (Temp)" <- w653
      }
    }
    n259 = call "Time Delay"("error in (no error)"=w438, "Delay Time (s)"=w386) -> ()  [unwired: 9 in, 1 out]
  }
  n260 = Initialize Array(0.0, 1000) -> (→"Baseline":dbl[])
  n261 = Initialize Array(0.0 ("number"), 1000) -> (→"Fit":dbl[])
  n262 = Initialize Array(0.0, 1000) -> (→"Fit X values":dbl[])
  n263 = Initialize Array(0.0, 1000) -> (→"Zeroed Array":dbl[])
  n264 = Get Date/Time String(seconds (now)=w17, want seconds? (F)=TRUE) -> (date string=w16:string, time string=w14:string)  [unwired: 1 in]
  n265 = Concatenate Strings(w16, " ", w14) -> (→"VI Start Time":string)
